vi "getImageAnalysis.vi"(8 "error in (no error)":errorcluster, 11 "FileSystem in":refnum<class "FileSystem.lvclass">) -> (0 "error out":errorcluster, 2 "ImageAnalysis":path, 3 "FileSystem out":refnum<class "FileSystem.lvclass">)   [LabVIEW 2009, in "Tools.lvlib" / "Filing.lvlib" / "FileSystem.lvclass"]
uses:
  FileSystem.lvclass
  FileSystem.lvclass/FileSystem.ctl
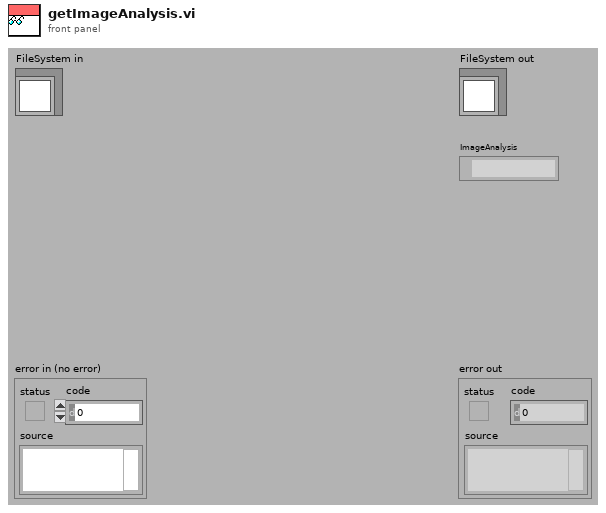
[diagram p1: front panel]
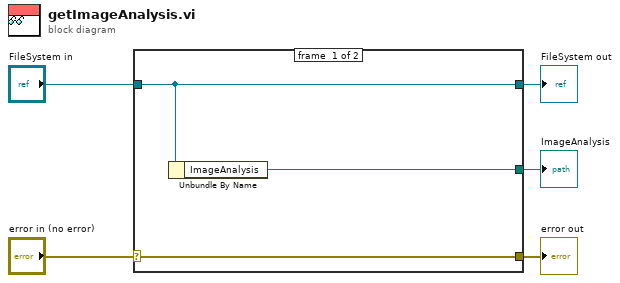
[diagram p0: block diagram]
diagram:
  n1 = case shown="No Error" "error in (no error)" {
    selector: "error in (no error)" -> [w8 w9]
    tunnel: [w8 w9] -> w4
    tunnel: [w7 w10] -> w2
    tunnel: "FileSystem in" -> [w7 w10]
    tunnel: [w6 _] -> w1
    frame #0 {
      n2 = Unbundle By Name(w7) -> ("ImageAnalysis"=w6:path)
    }
    frame #1 {
    }
  }
  "error out" <- w4
  "FileSystem out" <- w2
  "ImageAnalysis" <- w1
